vi "Find Broken VIs in a Folder.vi"(8 "error in (no error)":errorcluster, 11 "Directory Path":path) -> (0 "error out":errorcluster, 3 "Broken VIs":path[](array[path]))   [LabVIEW 2016, in "SLL Scripting.lvlib"]
doc: "This VI can be used to find the list of broken VIs in a folder. This also returns VIs which are of higher LabVIEW version than the currently used LabVIEW version."
uses:
  SLL Scripting.lvlib
panel:
  out "Progress":i32
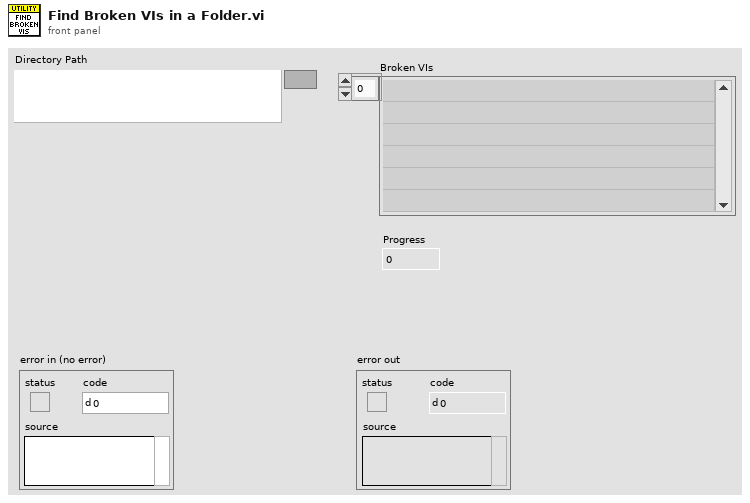
[diagram p1: front panel]
types:
  T1 = enum32{"Bad", "Idle", "Run top level", "Running"}
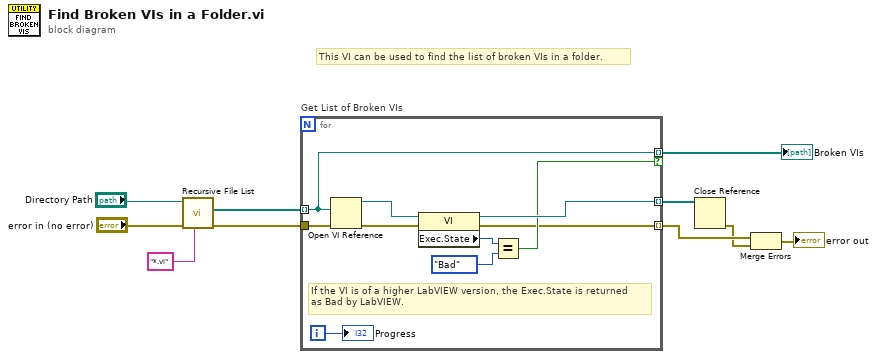
[diagram p0: block diagram]
diagram:
  # "This VI can be used to find the list of broken VIs in a folder."
  n1 = call <vilib>:"Recursive File List.vi"("pattern"="*.vi", "error in (no error)"="error in (no error)", "Folder Path"="Directory Path") -> ("error out"=w4:errorcluster, "All Files in Dir"=w7:path[])  [unwired: 4 in, 3 out]
  n2 = for "Get List of Broken VIs" {
    tunnel: [w17] -> w10 mode=indexing
    tunnel: w7 -> [w16] mode=indexing
    tunnel: [w16] -> w6 mode=indexing if=w15
    tunnel: w4 -> [w14]
    tunnel: [w12] -> w3 mode=indexing
    i -> [w11]
    # "If the VI is of a higher LabVIEW version, the Exec.State is returned\nas Bad by LabVIEW."
    n3 = Open VI Reference(vi path=w16, error in (no error)=w14) -> (vi reference=w20:refnum<vi>, error out=w13:errorcluster)  [unwired: 4 in]
    n4 = property class="VI"(reference=w20, error in=w13) -> (reference out=w17:refnum<vi>, error out=w12:errorcluster, "Exec.State"=w19:T1)
    n5 = Equal?(x=w19, y=T1."Bad" ("Execution:State")) -> (x = y?=w15:bool)
    "Progress" <- w11
  }
  "Broken VIs" <- w6
  n6 = Close Reference(reference=w10) -> (error out=w2:errorcluster)  [unwired: 1 in]
  n7 = Merge Errors(w3, w2) -> (→"error out":errorcluster)
